vi "Sig_Digital_Create.vi"(0 "reference in":refnum<class "Sig_Digital.lvclass">, 1 "DefaultConfig":T1, 5 "error in (no error)":errorcluster) -> (14 "reference out":refnum<class "Sig_Digital.lvclass">, 19 "error out":errorcluster)   [LabVIEW 2019, in "Sig_Digital.lvclass"]
doc: "Constructor."
uses:
  Sig_Digital.lvclass
  TypeDef/Config_Digital.ctl
  Sig_Digital.lvclass/Sig_Digital.ctl
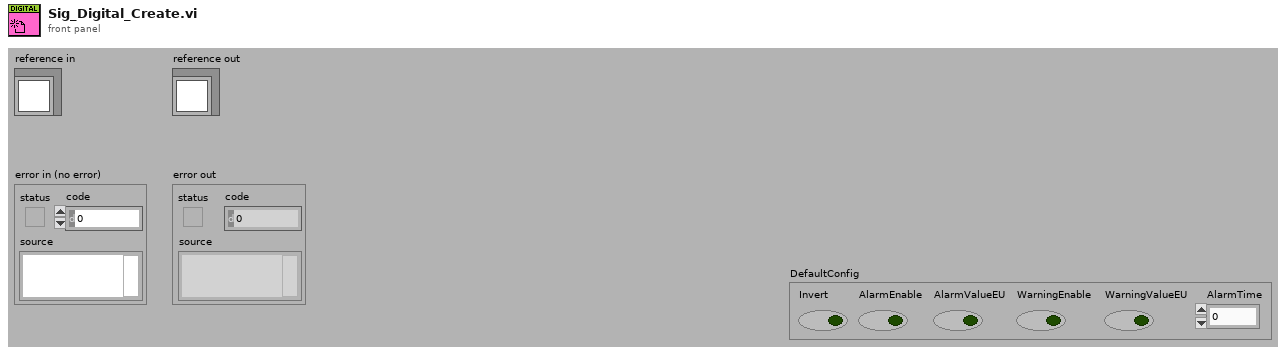
[diagram p1: front panel]
types:
  T1 = typedef "Config_Digital.ctl" = cluster{"Invert":bool, "AlarmEnable":bool, "AlarmValueEU":bool, "WarningEnable":bool, "WarningValueEU":bool, "AlarmTime":dbl}
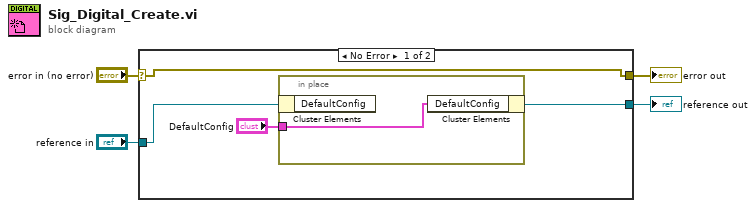
[diagram p0: block diagram]
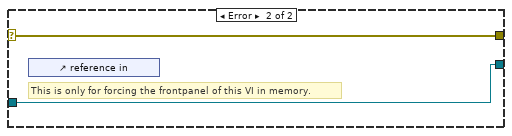
[diagram p2: hidden frame]
diagram:
  n1 = case shown="No Error" "error in (no error)" {
    selector: "error in (no error)" -> [w8 w11]
    tunnel: [w8 w11] -> w3
    tunnel: [w6 w10] -> w1
    tunnel: "reference in" -> [w5 w10]
    frame No Error {
      n2 = in-place {
        in-place-border: "DefaultConfig" -> [w9]
        n3 = in-place-cluster #1(w5) -> ()  [unwired: 1 out]
        n4 = in-place-cluster #1("DefaultConfig"=w9) -> (w6:refnum<class "Sig_Digital.lvclass">)
      }
    }
    frame Error {
      # "This is only for forcing the frontpanel of this VI in memory."
      n5 = control-ref of="reference in"() -> ()  [unwired: 1 out]
    }
  }
  "error out" <- w3
  "reference out" <- w1
